vi "WriteToSI.vi"(9 "Custom ROI":string, 11 "Refnum in":refnum<vi>) -> (0 "error out":errorcluster, 3 "Refnum out":refnum<vi>)   [LabVIEW 2015]
uses:
  SIcamera_Globals.vi
panel:
  in  "SI camera info":T1={"Observer Name"="", "object name"="", "File name base"="Red", "Camera Color"="", "Exp type tab"=enum."Object", "Number of Exp"=0.0, "Exp time"=0.0, "CCD Readout Speed"=5, "CCD ROI Mode"=10, "Hg(Ar)"=FALSE, "Cu"=FALSE, "Ne"=FALSE, "Bulb"=FALSE, "Ar"=FALSE, "Quartz"=FALSE, "Quartz Percent"=0.0, "Fe"=FALSE, "Notes"="", "Target Number"="", "Cam Focus"=0.0} {"CCD Readout Speed" items=["750 kHz, ATTN 0", "750 kHz, ATTN 2", "344 kHz, ATTN 0", "344 kHz, ATTN 3", "100 kHz, ATTN 2", "100 kHz, ATTN 3"]; "CCD ROI Mode" items=["Imaging, 1x1  "=0, "Imaging, 2x2"=1, "Imaging, 3x3"=2, "Spectroscopic, 1x1"=3, "Spectroscopic, 2x2"=4, "Spectroscopic, 3x3"=5, "MOS, 1x1"=11, "MOS, 2x2"=12, "MOS, 3x3"=13, "Slicer"=6, "Spectroscopic, ZZ Ceti"=14, "Slit Imaging/Alignment"=7, "MOS Imaging/Alignment"=10, "Set user-defined ROI..."=21, "Custom Mode"=9]}
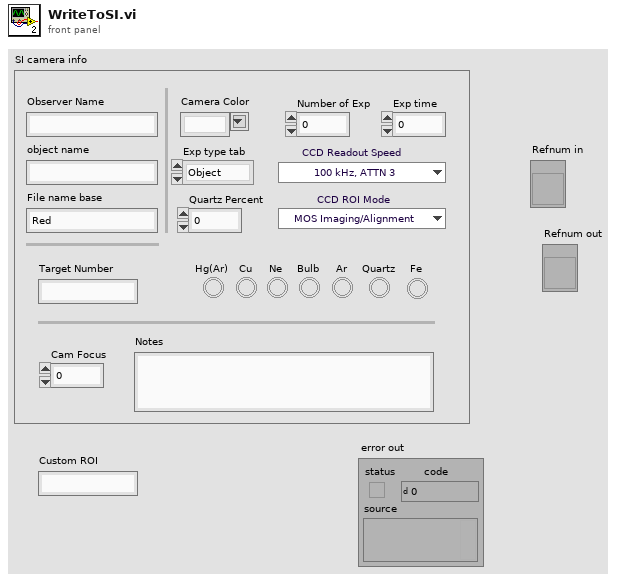
[diagram p1: front panel]
types:
  T1 = cluster{"Observer Name":string, "object name":string, "File name base":string, "Camera Color":string, "Exp type tab":enum16{"Object", "Flat", "Comp", "Dark", "Zero"}, "Number of Exp":dbl, "Exp time":dbl, "CCD Readout Speed":u8, "CCD ROI Mode":u16, "Hg(Ar)":bool, "Cu":bool, "Ne":bool, "Bulb":bool, "Ar":bool, "Quartz":bool, "Quartz Percent":dbl, "Fe":bool, "Notes":string, "Target Number":string, "Cam Focus":dbl}
  T2 = cluster{"ROI Mode":refnum<vi>, "RO Speed":refnum<vi>, "File name":refnum<vi>, "Exp time":refnum<vi>, "Start exp":refnum<vi>, "num exp":refnum<vi>, "cam color":refnum<vi>, "Exp tab":refnum<vi>, "notes":refnum<vi>, "observer name":refnum<vi>, "object name":refnum<vi>, "Ar":refnum<vi>, "Bulb":refnum<vi>, "Fe":refnum<vi>, "Hg(Ar)":refnum<vi>, "Cu":refnum<vi>, "Ne":refnum<vi>, "Quartz":refnum<vi>, "Quartz percent":refnum<vi>, "flat exp":refnum<vi>, "comp exp":refnum<vi>, "dark exp":refnum<vi>, "zero exp":refnum<vi>}
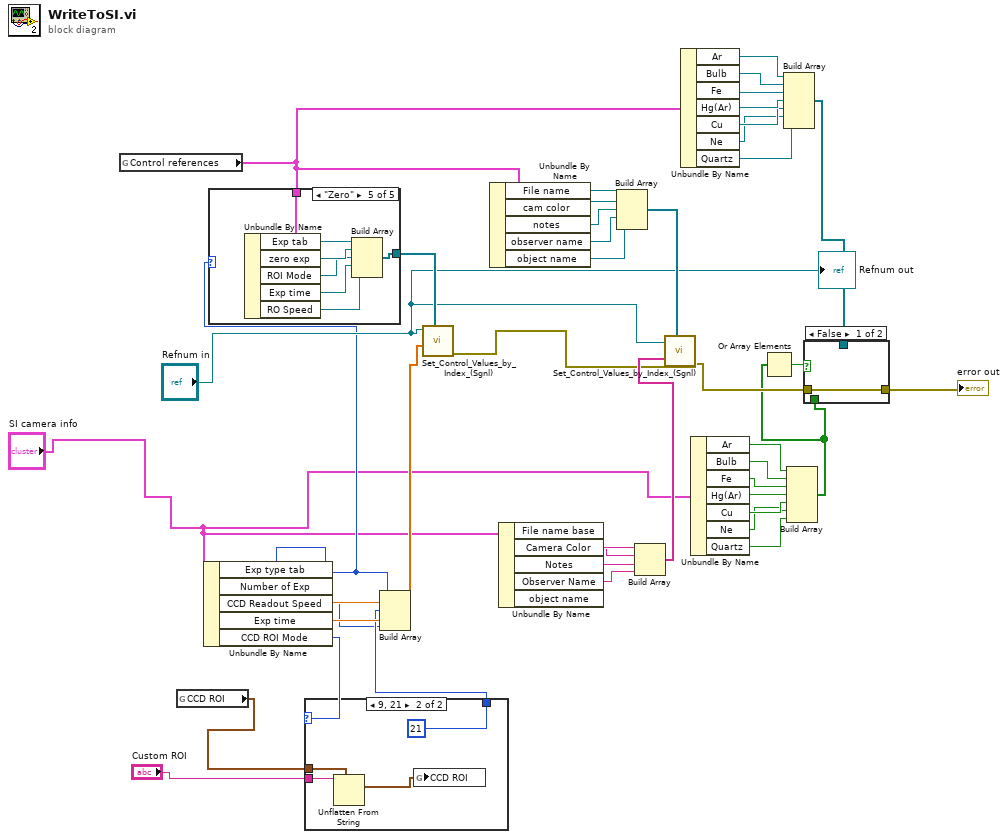
[diagram p0: block diagram]
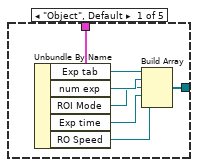
[diagram p2: hidden frame]
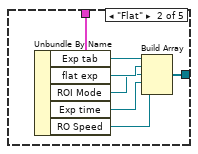
[diagram p3: hidden frame]
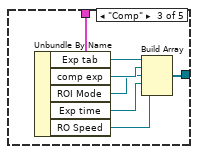
[diagram p4: hidden frame]
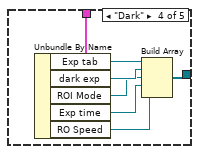
[diagram p5: hidden frame]
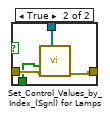
[diagram p7: hidden frame]
diagram:
  n1 = global read "SIcamera_Globals.vi" "Control references"() -> (w28:T2)
  n2 = global read "SIcamera_Globals.vi" "CCD ROI"() -> (w3:cluster{i32, i32, i32, i32, i32, i32})
  n3 = Unbundle By Name("SI camera info") -> ("Exp type tab"=w2:enum16{"Object", "Flat", "Comp", "Dark", "Zero"}, "Number of Exp"=w44:dbl, "CCD Readout Speed"=w4:u8, "Exp time"=w43:dbl, "CCD ROI Mode"=w7:u16)
  n4 = case shown="\"Zero\"" w2 {
    tunnel: [w45 w53 w59 w66 w73] -> w30
    tunnel: w28 -> [w46 w52 w60 w67 w74]
    frame "Object", Default {
      n5 = Unbundle By Name(w46) -> ("Exp tab"=w47:refnum<vi>, "num exp"=w51:refnum<vi>, "ROI Mode"=w50:refnum<vi>, "Exp time"=w49:refnum<vi>, "RO Speed"=w48:refnum<vi>)
      n6 = Build Array(w47, w51, w50, w49, w48) -> (w45:refnum<vi>[])
    }
    frame "Flat" {
      n7 = Unbundle By Name(w52) -> ("Exp tab"=w54:refnum<vi>, "flat exp"=w58:refnum<vi>, "ROI Mode"=w57:refnum<vi>, "Exp time"=w56:refnum<vi>, "RO Speed"=w55:refnum<vi>)
      n8 = Build Array(w54, w58, w57, w56, w55) -> (w53:refnum<vi>[])
    }
    frame "Comp" {
      n9 = Unbundle By Name(w60) -> ("Exp tab"=w61:refnum<vi>, "comp exp"=w65:refnum<vi>, "ROI Mode"=w64:refnum<vi>, "Exp time"=w63:refnum<vi>, "RO Speed"=w62:refnum<vi>)
      n10 = Build Array(w61, w65, w64, w63, w62) -> (w59:refnum<vi>[])
    }
    frame "Dark" {
      n11 = Unbundle By Name(w67) -> ("Exp tab"=w68:refnum<vi>, "dark exp"=w72:refnum<vi>, "ROI Mode"=w71:refnum<vi>, "Exp time"=w70:refnum<vi>, "RO Speed"=w69:refnum<vi>)
      n12 = Build Array(w68, w72, w71, w70, w69) -> (w66:refnum<vi>[])
    }
    frame "Zero" {
      n13 = Unbundle By Name(w74) -> ("Exp tab"=w75:refnum<vi>, "zero exp"=w79:refnum<vi>, "ROI Mode"=w78:refnum<vi>, "Exp time"=w77:refnum<vi>, "RO Speed"=w76:refnum<vi>)
      n14 = Build Array(w75, w79, w78, w77, w76) -> (w73:refnum<vi>[])
    }
  }
  n15 = case shown="9, 21" w7 {
    selector: w7 -> [w80 _]
    tunnel: [w80 21] -> w5
    tunnel: "Custom ROI" -> [_ w83]
    tunnel: w3 -> [_ w82]
    frame 0, Default {
    }
    frame 9, 21 {
      n16 = Unflatten From String(type=w82, binary string=w83) -> (value=w81:cluster{i32, i32, i32, i32, i32, i32})  [unwired: 3 in, 2 out]
      n17 = global write "SIcamera_Globals.vi" "CCD ROI"(w81) -> ()
    }
  }
  n18 = Build Array(w2, w44, w5, w43, w4) -> (w38:dbl[])
  n19 = call "Set_Control_Values_by_Index_(Sgnl).vi"("Control References"=w30, "appended array"=w38, "VI Refnum"="Refnum in") -> ("error out"=w36:errorcluster)  [unwired: 8 in]
  n20 = Unbundle By Name(w28) -> ("File name"=w35:refnum<vi>, "cam color"=w34:refnum<vi>, "notes"=w33:refnum<vi>, "observer name"=w32:refnum<vi>, "object name"=w31:refnum<vi>)
  n21 = Unbundle By Name("SI camera info") -> ("File name base"=w42:string, "Camera Color"=w41:string, "Notes"=w40:string, "Observer Name"=w39:string)  [unwired: 1 out]
  n22 = Build Array(w35, w34, w33, w32, w31) -> (w29:refnum<vi>[])
  n23 = Build Array(w42, w41, w40, w39) -> (w37:string[])
  n24 = call "Set_Control_Values_by_Index_(Sgnl).vi"("Control References"=w29, "error in (no error)"=w36, "appended array"=w37, "VI Refnum"="Refnum in") -> ("error out"=w12:errorcluster)  [unwired: 7 in]
  n25 = Unbundle By Name(w28) -> ("Ar"=w27:refnum<vi>, "Bulb"=w26:refnum<vi>, "Fe"=w25:refnum<vi>, "Hg(Ar)"=w24:refnum<vi>, "Cu"=w23:refnum<vi>, "Ne"=w22:refnum<vi>, "Quartz"=w21:refnum<vi>)
  n26 = Unbundle By Name("SI camera info") -> ("Ar"=w20:bool, "Bulb"=w19:bool, "Fe"=w18:bool, "Hg(Ar)"=w17:bool, "Cu"=w16:bool, "Ne"=w15:bool, "Quartz"=w14:bool)
  n27 = Build Array(w27, w26, w25, w24, w23, w22, w21) -> (w11:refnum<vi>[])
  n28 = Build Array(w20, w19, w18, w17, w16, w15, w14) -> (w8:bool[])
  n29 = Or Array Elements(Boolean array=w8) -> (logical OR=w9:bool)
  n30 = case shown="False" w9 {
    tunnel: [w85 w89] -> w13
    tunnel: w12 -> [w85 w88]
    tunnel: w8 -> [_ w87]
    tunnel: w11 -> [_ w86]
    frame False {
    }
    frame True {
      n31 = call "Set_Control_Values_by_Index_(Sgnl) for Lamps.vi"("Control References"=w86, "error in (no error)"=w88, "appended array"=w87) -> ("error out"=w89:errorcluster)  [unwired: 8 in]
    }
  }
  "error out" <- w13
  "Refnum out" <- "Refnum in"
